vi "Read ModuleWidth.vi"(8 "error in (no error)":errorcluster, 11 "Linear Barcode in":refnum<class "Linear Barcode.lvclass">) -> (0 "error out":errorcluster, 2 "ModuleWidth":u8=1, 3 "Linear Barcode out":refnum<class "Linear Barcode.lvclass">)   [LabVIEW 2013, in "BarCodes.lvlib" / "Linear Barcode.lvclass"]
uses:
  Linear Barcode.lvclass
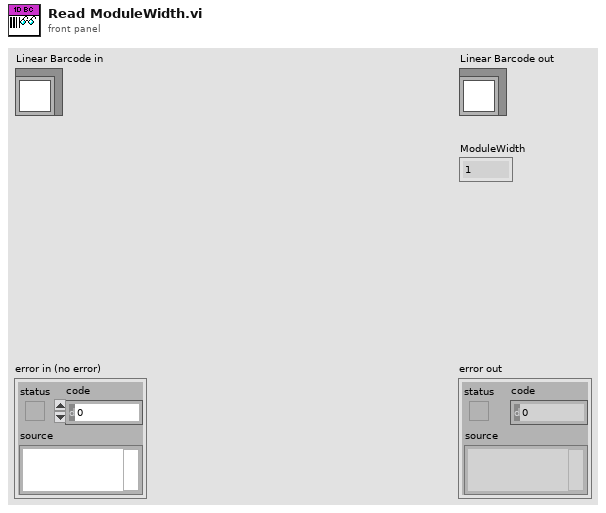
[diagram p1: front panel]
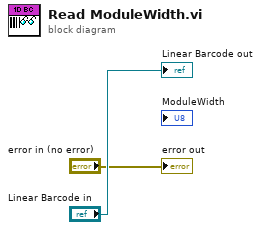
[diagram p0: block diagram]
diagram:
  "error out" <- "error in (no error)"
  "Linear Barcode out" <- "Linear Barcode in"
